vi "Error detection and correction.vi"() -> ()   [LabVIEW 2014]
uses:
  <vilib>/Analysis/7linalg.llb/Create Special Real Matrix.vi
  <vilib>/Analysis/Matrix/Numeric/Conversions/Matrix To Array - RM.vi
  <vilib>/Analysis/NI_AALPro.lvlib
  <vilib>/Analysis/Matrix/NI_Matrix.lvlib
panel:
  out "Identity matrix(n) 2":dbl[][](array[numeric])
  out "R":bool[](array[boolean])
  out "Corrected code word":bool[](array[boolean])
  out "Error bit":dbl
  out "Condition":string
  out "SYNDROME":i32[](array[numeric])
  in  "C":bool[](array[boolean])
  out "codewords":i32[][](array[numeric])
  out "messages":i16[][](array[numeric])
  out "Parity check matrix Ht":dbl[][](array[numeric])
  out "Generator matrix G":dbl[][](array[numeric])
  in  "Parity matrix P":dbl[][](array[numeric])
  in  "k":dbl
  in  "n":dbl
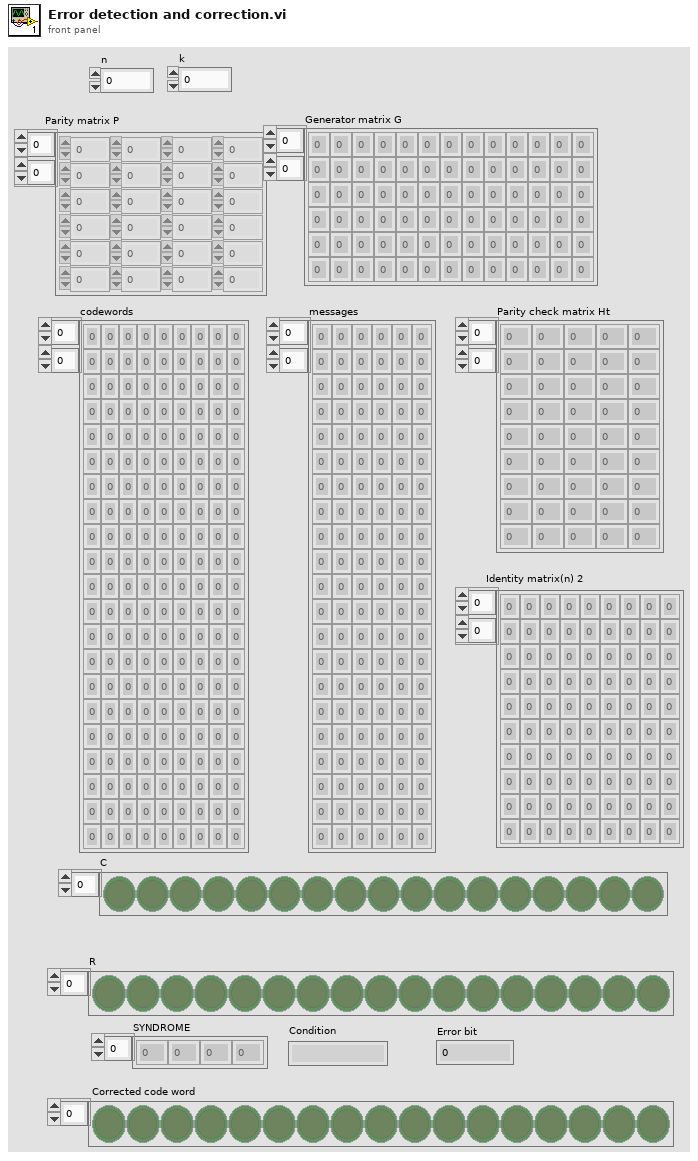
[diagram p1: front panel]
types:
  T1 = typedef "NI_Matrix.lvlib/RealMatrix.ctl" = dbl[][]
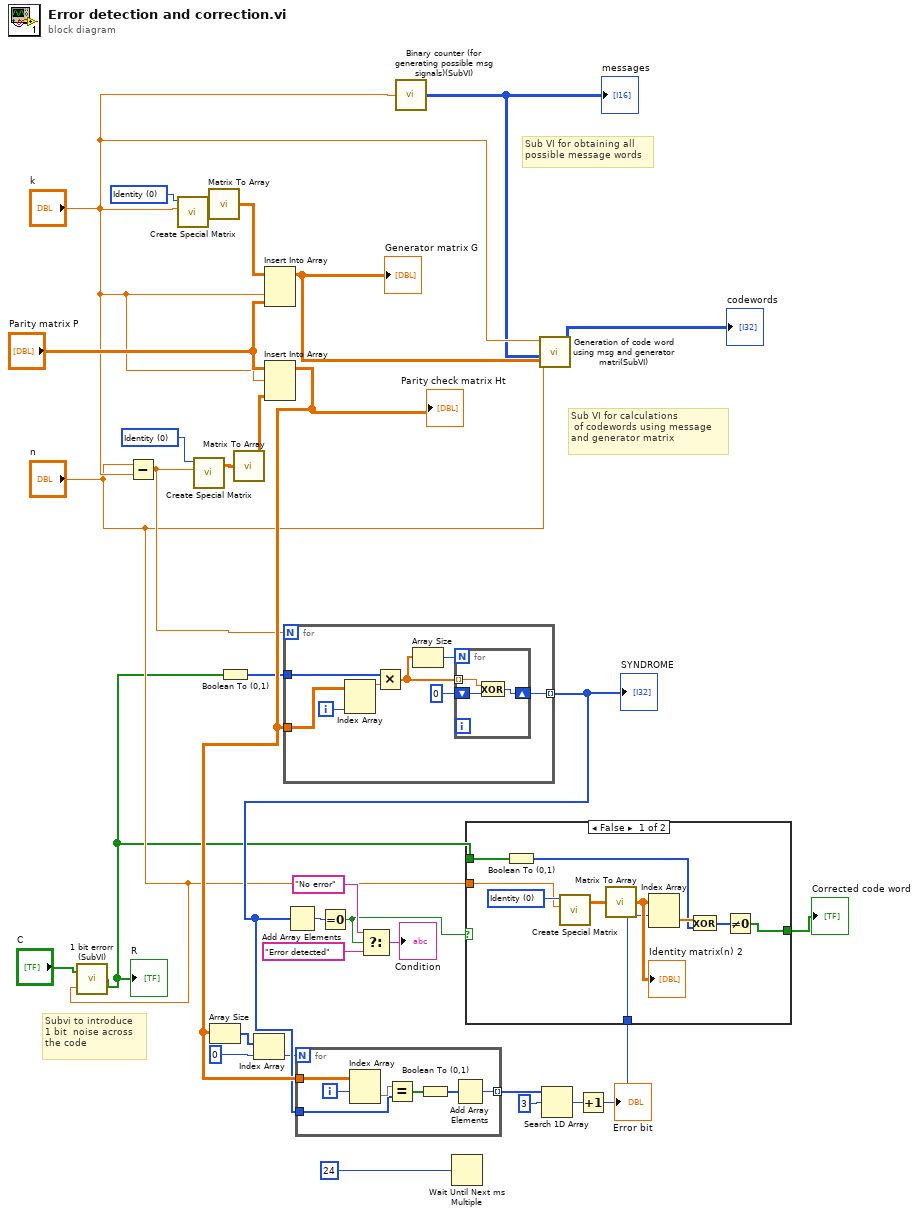
[diagram p0: block diagram]
diagram:
  w30 = 0 items=["Identity", "Diagonal", "Toeplitz", "Vandermonde", "Companion", "Hankel", "Hadamard", "Wilkinson", "Hilbert", "Inverse Hilbert", "Rosser", "Pascal"] ("matrix type")
  w32 = 0 items=["Identity", "Diagonal", "Toeplitz", "Vandermonde", "Companion", "Hankel", "Hadamard", "Wilkinson", "Hilbert", "Inverse Hilbert", "Rosser", "Pascal"] ("matrix type")
  # "Subvi to introduce \n1 bit  noise across \nthe code"
  # "Sub VI for obtaining all \npossible message words"
  # "Sub VI for calculations\n of codewords using message\nand generator matrix"
  n1 = call "1 bit errorr (SubVI).vi"("Numeric"="n", "R in"="C") -> ("R out"=w2:bool[])
  "R" <- w2
  n2 = Subtract(x="n", y="k") -> (x-y=w7:dbl)
  n3 = call-poly <vilib>:"Create Special Matrix.vi"("matrix type"=w30, "matrix size"="k") -> ("Special Matrix"=w29:T1)  [unwired: 3 in, 1 out]
  n4 = call-poly <vilib>:"Create Special Matrix.vi"("matrix type"=w32, "matrix size"=w7) -> ("Special Matrix"=w31:T1)  [unwired: 3 in, 1 out]
  n5 = call-poly <vilib>:"Matrix To Array.vi"("Real Matrix"=w29) -> ("Real 2D Array"=w28:dbl[][])
  n6 = Boolean To (0,1)(Boolean=w2) -> (0, 1=w4:i16[])
  n7 = call-poly <vilib>:"Matrix To Array.vi"("Real Matrix"=w31) -> ("Real 2D Array"=w26:dbl[][])
  n8 = Insert Into Array(array=w28, index (col)="k", new element="Parity matrix P") -> (w25:dbl[][])  [unwired: 1 in]
  "Generator matrix G" <- w25
  n9 = Insert Into Array(array="Parity matrix P", index (row)="k", new element=w26) -> (w12:dbl[][])  [unwired: 1 in]
  "Parity check matrix Ht" <- w12
  n10 = Array Size(array=w12) -> (size(s)=w17:i32[])
  n11 = Index Array(array=w17, index=0) -> (element=w10:i32)
  n12 = for {
    N: w7 -> [_]
    tunnel: w12 -> [w40]
    tunnel: w4 -> [w38]
    tunnel: [w33] -> w11 mode=indexing
    i -> [w34]
    n13 = Index Array(array=w40, index (col)=w34) -> (element=w37:dbl[])  [unwired: 1 in]
    n14 = Multiply(x=w38, y=w37) -> (x*y=w35:dbl[])
    n15 = Array Size(array=w35) -> (size(s)=w36:i32)
    n16 = for {
      N: w36 -> [_]
      tunnel: w35 -> [w41] mode=indexing
      shift-right: [w42] -> w33
      shift-left: 0 -> [w43]
      n17 = Exclusive Or(1:w43, 2:w41) -> (0:w42:i32)
    }
  }
  "SYNDROME" <- w11
  n18 = Add Array Elements(numeric array=w11) -> (sum=w18:i32)
  n19 = for {
    N: w10 -> [_]
    tunnel: w11 -> [w44]
    tunnel: w12 -> [w50]
    tunnel: [w47] -> w15 mode=indexing
    i -> [w48]
    n20 = Index Array(array=w50, index (row)=w48) -> (element=w49:dbl[])  [unwired: 1 in]
    n21 = Equal?(x=w49, y=w44) -> (x = y?=w46:bool[])
    n22 = Boolean To (0,1)(Boolean=w46) -> (0, 1=w45:i16[])
    n23 = Add Array Elements(numeric array=w45) -> (sum=w47:i16)
  }
  n24 = Equal To 0?(x=w18) -> (x = 0?=w3:bool)
  n25 = Select(t="No error", s=w3, f="Error detected") -> (s? t:f=→"Condition":string)
  n26 = call "Binary counter (for generating possible msg signals)(SubVI).vi"("k"="k") -> ("msg words"=w23:i16[][])
  "messages" <- w23
  n27 = Wait Until Next ms Multiple(millisecond multiple=u32 24) -> ()  [unwired: 1 out]
  n28 = call "Generation of code word using msg and generator matri(SubVI).vi"("G in"=w25, "messages in"=w23, "n"="n", "k"="k") -> ("Array"=→"codewords":i32[][])  [unwired: 7 in]
  n29 = Search 1D Array(1D array=w15, element=i16 3) -> (index of element=w9:i32)  [unwired: 1 in]
  n30 = case shown="False" w3 {
    tunnel: w9 -> [w55 _]
    tunnel: [w53 w61] -> w8
    tunnel: "n" -> [w54 _]
    tunnel: w2 -> [w52 w61]
    frame False {
      w60 = 0 items=["Identity", "Diagonal", "Toeplitz", "Vandermonde", "Companion", "Hankel", "Hadamard", "Wilkinson", "Hilbert", "Inverse Hilbert", "Rosser", "Pascal"] ("matrix type")
      n31 = Boolean To (0,1)(Boolean=w52) -> (0, 1=w51:i16[])
      n32 = call-poly <vilib>:"Create Special Matrix.vi"("matrix type"=w60, "matrix size"=w54) -> ("Special Matrix"=w59:T1)  [unwired: 3 in, 1 out]
      n33 = call-poly <vilib>:"Matrix To Array.vi"("Real Matrix"=w59) -> ("Real 2D Array"=w58:dbl[][])
      "Identity matrix(n) 2" <- w58
      n34 = Index Array(array=w58, index (row)=w55) -> (element=w57:dbl[])  [unwired: 1 in]
      n35 = Exclusive Or(1:w51, 2:w57) -> (0:w56:i32[])
      n36 = Not Equal To 0?(x=w56) -> (x != 0?=w53:bool[])
    }
    frame True {
    }
  }
  "Corrected code word" <- w8
  n37 = Increment(x=w9) -> (x+1=→"Error bit":i32)
